vi "AddArrayCtls.vi"(8 "error IO In":errorcluster, 11 "CtlLookup In":T1) -> (0 "error IO":errorcluster, 3 "CtlLookup Out":T1)   [LabVIEW 2020, in "CtlReferences.lvlib" / "CtlReferences.lvclass"]
doc: "Add all cluster (and subcluster) element control refs\nto the DVR ctl storage. -- Cluster names are specified by ClusterName.ControlName"
uses:
  CtlReferences.lvclass
  TypeDefs/CtlLookup.ctl
  CtlReferences.lvclass/CtlReferences.ctl
  AddControl.vi
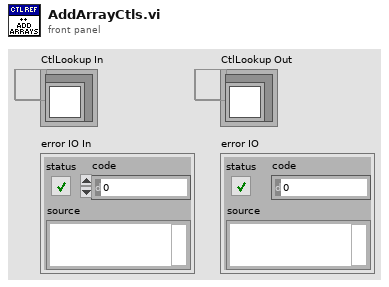
[diagram p1: front panel]
types:
  T1 = typedef "CtlReferences.lvlib/CtlReferences.lvclass/CtlLookup.ctl" = refnum<data-value>
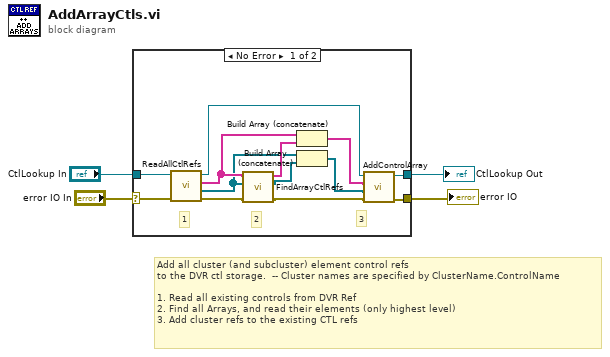
[diagram p0: block diagram]
diagram:
  # "Add all cluster (and subcluster) element control refs\nto the DVR ctl storage.  -- Cluster names are specified by ClusterName.ControlName\n\n1. Read all existing controls from DVR Ref\n2. Find all Arrays, and read their elements (only highest level)\n3. Add cluster refs to the existing CTL refs"
  n1 = case shown="No Error" "error IO In" {
    selector: "error IO In" -> [w16 w19]
    tunnel: "CtlLookup In" -> [w17 w18]
    tunnel: [w14 w18] -> w2
    tunnel: [w15 w19] -> w1
    frame No Error {
      # "3"
      # "2"
      # "1"
      n2 = call "ReadAllCtlRefs.vi"("error in (no error)"=w16, "CtlLookup In"=w17) -> ("error out"=w9:errorcluster, "CtlRef Array"=w5:refnum<vi>[], "CtlName Array"=w6:string[], "CtlLookup Out"=w13:T1)  [unwired: 6 in]
      n3 = call "FindArrayCtlRefs.vi"("error in (no error)"=w9, "CLT Ref Array"=w5, "CTL Name Array"=w6) -> ("error out"=w10:errorcluster, "Cluster CTL Array"=w7:refnum<vi>[], "Cluster CTL Name Array"=w8:string[])  [unwired: 6 in]
      n4 = Build Array (concatenate)(w6, w8) -> (w12:string[])
      n5 = Build Array (concatenate)(w5, w7) -> (w11:refnum<vi>[])
      n6 = call "AddControlArray.vi"("error in (no error)"=w10, "CtlRef Array"=w11, "CtlLabel Array"=w12, "CtlLookup In"=w13) -> ("error out"=w15:errorcluster, "CtlLookup Out"=w14:T1)  [unwired: 6 in]
    }
    frame Error {
    }
  }
  "error IO" <- w1
  "CtlLookup Out" <- w2
